vi "PBKDF2-SHA-256 hash.vi"(7 "PBKDF2 hash type":T1, 8 "Key Length":i32=32, 9 "Iterations":i32=100, 10 "Salt":string="salt123", 11 "Secret":string="secret") -> (3 "Hash string":string="EX1Y3Q9BMM2oGLxsGqDgFeuqtPMf7Wz8Lh6PotZ62ho=")   [LabVIEW 2020, in "wamplv.lvlib" / "WampCraAuthenticator.lvclass"]
uses:
  WampCraAuthenticator.lvclass
  PBKDF2 hash type.ctl
  Utils/Base64 Encode.vi
  Utils/Utils.lvclass
  HashLib/HashLib.lvclass
  wamplv.lvlib
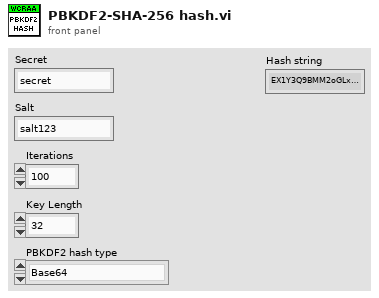
[diagram p1: front panel]
types:
  T1 = typedef "wamplv.lvlib/PBKDF2 hash type.ctl" = enum8{"Base64", "Hex string, lower case", "Hex string, upper case", "Direct to string cast"}
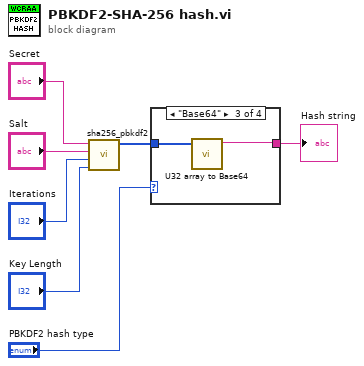
[diagram p0: block diagram]
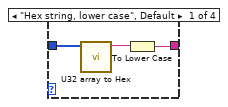
[diagram p2: hidden frame]
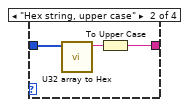
[diagram p3: hidden frame]
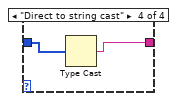
[diagram p4: hidden frame]
diagram:
  n1 = call "sha256_pbkdf2.vi"("dkLen (32octets=sha256)"="Key Length", "iterations"="Iterations", "salt"="Salt", "password"="Secret") -> ("sha-256"=w3:u32[])  [unwired: 7 in]
  n2 = case shown="\"Base64\"" "PBKDF2 hash type" {
    tunnel: w3 -> [w10 w13 w15 w16]
    tunnel: [w8 w11 w14 w17] -> w2
    frame "Hex string, lower case", Default {
      n3 = call "U32 array to Hex.vi"("Array"=w10) -> ("Hex string"=w9:string)  [unwired: 10 in]
      n4 = To Lower Case(string=w9) -> (all lower case string=w8:string)
    }
    frame "Hex string, upper case" {
      n5 = call "U32 array to Hex.vi"("Array"=w13) -> ("Hex string"=w12:string)  [unwired: 10 in]
      n6 = To Upper Case(1:w12) -> (0:w11:string)
    }
    frame "Base64" {
      n7 = call "U32 array to Base64.vi"("Array"=w15) -> ("Base64 sring out"=w14:string)  [unwired: 10 in]
    }
    frame "Direct to string cast" {
      n8 = Type Cast(x=w16) -> (*(type *) &x=w17:string)  [unwired: 1 in]
    }
  }
  "Hash string" <- w2
